vi "S4GUI_003.vi"(7 "Tab ObsEng":enum32{"Obs", "CCD modes", "Guider", "Eng"}(tab)) -> ()   [LabVIEW 2018] (continued)
                n3107 = call-dynamic "Write State Machine.vi"("error in (no error)"=w6764, "State Machine.lvclass"=w6763, "Device in"=w6747) -> ("error out"=w6744:errorcluster, "Device out"=w6746:refnum<class "Channel.lvclass">)  [unwired: 7 in]
              }
            }
            n3108 = case shown="True" w6438 {
              tunnel: w6496 -> [w6710 w6719]
              tunnel: w6495 -> [w6709 w6718]
              tunnel: [w6709 w6717] -> w6494
              tunnel: [w6710 w6716] -> w6493
              frame False {
              }
              frame True {
                n3109 = call-dynamic "Read State Machine.vi"("error in (no error)"=w6718, "Device in"=w6719) -> ("error out"=w6732:errorcluster, "State Machine.lvclass"=w6733:refnum<class "State Machine.lvclass">, "Device out"=w6720:refnum<class "Channel.lvclass">)  [unwired: 7 in]
                n3110 = call-dynamic "Read ref StatesQueue.vi"("error in (no error)"=w6732, "State Machine in"=w6733) -> ("error out"=w6730:errorcluster, "ref StatesQueue"=w6731:refnum<queue>, "State Machine out"=w6727:refnum<class "State Machine.lvclass">)  [unwired: 7 in]
                n3111 = Flush Queue(queue=w6731, error in (no error)=w6730) -> (queue out=w6729:refnum<queue>, error out=w6725:errorcluster)  [unwired: 1 out]
                n3112 = Enqueue Element(queue=w6729, element=u32 300 ("State"), error in (no error)=w6725) -> (queue out=w6714:refnum<queue>, error out=w6712:errorcluster)  [unwired: 1 in, 1 out]
                n3113 = Enqueue Element(queue=w6714, element=u32 305 ("State"), error in (no error)=w6712) -> (queue out=w6713:refnum<queue>, error out=w6711:errorcluster)  [unwired: 1 in, 1 out]
                n3114 = Enqueue Element(queue=w6713, element=u32 60 ("State"), error in (no error)=w6711) -> (queue out=w6728:refnum<queue>, error out=w6726:errorcluster)  [unwired: 1 in, 1 out]
                n3115 = call-dynamic "Write ref StatesQueue.vi"("error in (no error)"=w6726, "ref StatesQueue"=w6728, "State Machine in"=w6727) -> ("error out"=w6723:errorcluster, "State Machine out"=w6724:refnum<class "State Machine.lvclass">)  [unwired: 7 in]
                n3116 = call-dynamic "Write State.vi"("error in (no error)"=w6723, "State"=0, "State Machine in"=w6724) -> ("error out"=w6736:errorcluster, "State Machine out"=w6735:refnum<class "State Machine.lvclass">)  [unwired: 7 in]
                n3117 = call-dynamic "Write State Machine.vi"("error in (no error)"=w6736, "State Machine.lvclass"=w6735, "Device in"=w6720) -> ("error out"=w6717:errorcluster, "Device out"=w6716:refnum<class "Channel.lvclass">)  [unwired: 7 in]
              }
            }
            n3118 = case shown="True" w6439 {
              tunnel: w6446 -> [w6682 w6695]
              tunnel: w6445 -> [w6681 w6694]
              tunnel: [w6681 w6693] -> w6444
              tunnel: [w6682 w6692] -> w6443
              frame False {
              }
              frame True {
                n3119 = call-dynamic "Read State Machine.vi"("error in (no error)"=w6694, "Device in"=w6695) -> ("error out"=w6706:errorcluster, "State Machine.lvclass"=w6691:refnum<class "State Machine.lvclass">, "Device out"=w6696:refnum<class "Channel.lvclass">)  [unwired: 7 in]
                n3120 = call-dynamic "Read ref StatesQueue.vi"("error in (no error)"=w6706, "State Machine in"=w6691) -> ("error out"=w6704:errorcluster, "ref StatesQueue"=w6705:refnum<queue>, "State Machine out"=w6690:refnum<class "State Machine.lvclass">)  [unwired: 7 in]
                n3121 = Flush Queue(queue=w6705, error in (no error)=w6704) -> (queue out=w6703:refnum<queue>, error out=w6700:errorcluster)  [unwired: 1 out]
                n3122 = Enqueue Element(queue=w6703, element=u32 300 ("State"), error in (no error)=w6700) -> (queue out=w6686:refnum<queue>, error out=w6685:errorcluster)  [unwired: 1 in, 1 out]
                n3123 = Enqueue Element(queue=w6686, element=u32 305 ("State"), error in (no error)=w6685) -> (queue out=w6684:refnum<queue>, error out=w6683:errorcluster)  [unwired: 1 in, 1 out]
                n3124 = Enqueue Element(queue=w6684, element=u32 60 ("State"), error in (no error)=w6683) -> (queue out=w6702:refnum<queue>, error out=w6701:errorcluster)  [unwired: 1 in, 1 out]
                n3125 = call-dynamic "Write ref StatesQueue.vi"("error in (no error)"=w6701, "ref StatesQueue"=w6702, "State Machine in"=w6690) -> ("error out"=w6699:errorcluster, "State Machine out"=w6689:refnum<class "State Machine.lvclass">)  [unwired: 7 in]
                n3126 = call-dynamic "Write State.vi"("error in (no error)"=w6699, "State"=0, "State Machine in"=w6689) -> ("error out"=w6708:errorcluster, "State Machine out"=w6688:refnum<class "State Machine.lvclass">)  [unwired: 7 in]
                n3127 = call-dynamic "Write State Machine.vi"("error in (no error)"=w6708, "State Machine.lvclass"=w6688, "Device in"=w6696) -> ("error out"=w6693:errorcluster, "Device out"=w6692:refnum<class "Channel.lvclass">)  [unwired: 7 in]
              }
            }
            n3128 = call-dynamic "Write Channel.vi"("error in (no error)"=w6636, "Channel.lvclass"=w6637, "Acquisition in"=w6651) -> ("error out"=w6679:errorcluster, "Acquisition out"=w6680:refnum<class "Acquisition.lvclass">)  [unwired: 7 in]
            n3129 = call-dynamic "Write Channel.vi"("error in (no error)"=w6546, "Channel.lvclass"=w6548, "Acquisition in"=w6585) -> ("error out"=w6677:errorcluster, "Acquisition out"=w6678:refnum<class "Acquisition.lvclass">)  [unwired: 7 in]
            n3130 = call-dynamic "Write Channel.vi"("error in (no error)"=w6494, "Channel.lvclass"=w6493, "Acquisition in"=w6532) -> ("error out"=w6675:errorcluster, "Acquisition out"=w6676:refnum<class "Acquisition.lvclass">)  [unwired: 7 in]
            n3131 = call-dynamic "Write Channel.vi"("error in (no error)"=w6444, "Channel.lvclass"=w6443, "Acquisition in"=w6492) -> ("error out"=w6673:errorcluster, "Acquisition out"=w6674:refnum<class "Acquisition.lvclass">)  [unwired: 7 in]
          }
        }
        n3132 = call-dynamic "Write AcquisitionA.vi"("error in (no error)"=w5592, "Acquisition.lvclass"=w5593, "S4ACS_GUI in"=w5594) -> ("error out"=w5584:errorcluster, "S4ACS_GUI out"=w5588:refnum<class "S4GUI.lvclass">)  [unwired: 7 in]
        n3133 = call "Write AcquisitionB.vi"("error in (no error)"=w5589, "Acquisition.lvclass"=w5590, "S4ACS_GUI in"=w5588) -> ("error out"=w5583:errorcluster, "S4ACS_GUI out"=w5587:refnum<class "S4GUI.lvclass">)  [unwired: 7 in]
        n3134 = call-dynamic "Write AcquisitionC.vi"("error in (no error)"=w5578, "Acquisition.lvclass"=w5579, "S4ACS_GUI in"=w5587) -> ("error out"=w5582:errorcluster, "S4ACS_GUI out"=w5586:refnum<class "S4GUI.lvclass">)  [unwired: 7 in]
        n3135 = call-dynamic "Write AcquisitionD.vi"("error in (no error)"=w5576, "Acquisition.lvclass"=w5577, "S4ACS_GUI in"=w5586) -> ("error out"=w5581:errorcluster, "S4ACS_GUI out"=w5585:refnum<class "S4GUI.lvclass">)  [unwired: 7 in]
        n3136 = Merge Errors(w5584, w5583, w5582, w5581) -> (w5580:errorcluster)
        n3137 = call "Write cfg file.vi"("error in (no error)"=w5580, "cfg file"="lastsaved.cfg", "S4ACS_GUI in"=w5585) -> ("error out"=w5536:errorcluster, "S4ACS_GUI out"=w5537:refnum<class "S4GUI.lvclass">)  [unwired: 7 in]
        n3138 = disable-structure shown="Enabled" {
          disable-tunnel: w5537 -> [w5598 w5633]
          disable-tunnel: w5536 -> [w5597 w5632]
          disable-tunnel: [w5596 w5633] -> w5535
          disable-tunnel: [w5595 w5632] -> w5534
          frame Disabled {
            # "Este código passou para o evento \"Timeout\" (executa sempre)"
            # "1a vez FOTOM (F)"
            # "1a vez POLAR (F)"
            n3139 = call "Read Instrument.lvclass.vi"("error in (no error)"=w5597, "S4ACS_GUI in"=w5598) -> ("error out"=w5600:errorcluster, "Instrument.lvclass"=w5601:refnum<class "Instrument.lvclass">, "S4ACS_GUI out"=w5596:refnum<class "S4GUI.lvclass">)  [unwired: 7 in]
            n3140 = call-dynamic "Read mode.vi"("error in (no error)"=w5600, "Instrument in"=w5601) -> ("error out"=w5595:errorcluster, "mode"=w5599:bool)  [unwired: 7 in, 1 out]
            n3141 = while {
              tunnel: w5599 -> [w5606]
              shift-right: [w5602] -> _
              shift-left: _ -> [w5605]
              shift-right: [w5603] -> _
              shift-left: _ -> [w5604]
              stop <- TRUE stop-if-true
              # "Valores default para procedimento\nde ajuste de foco do telescópio"
              n3142 = case shown="True" w5606 {
                tunnel: w5605 -> [w5608 w5623]
                tunnel: [w5609 w5622] -> w5602
                tunnel: w5604 -> [w5611 w5621]
                tunnel: [w5610 w5620] -> w5603
                frame True {
                  # "polarimetria"
                  n3143 = case shown="False" w5611 {
                    selector: w5611 -> [w5615 w5619]
                    tunnel: [w5614 w5619] -> w5610
                    tunnel: [FALSE FALSE] -> w5609
                    tunnel: w5608 -> [_ _]
                    frame False {
                      w5612 = 12900
                      n3144 = local write "Start focus"(w5612) -> ()
                      n3145 = local write "Target focus"(w5612) -> ()
                      n3146 = local write "Step focus"(80) -> ()
                      n3147 = local write "#steps"(11) -> ()
                      n3148 = Not(x=w5615) -> (.not. x?=w5614:bool)
                    }
                    frame True {
                    }
                  }
                }
                frame False {
                  # "fotometria"
                  n3149 = case shown="False" w5623 {
                    selector: w5623 -> [w5626 w5631]
                    tunnel: [w5625 w5631] -> w5622
                    tunnel: w5621 -> [_ _]
                    tunnel: [FALSE FALSE] -> w5620
                    frame False {
                      w5624 = 13400
                      n3150 = local write "Start focus"(w5624) -> ()
                      n3151 = local write "Step focus"(100) -> ()
                      n3152 = local write "Target focus"(w5624) -> ()
                      n3153 = local write "#steps"(11) -> ()
                      n3154 = Not(x=w5626) -> (.not. x?=w5625:bool)
                    }
                    frame True {
                    }
                  }
                }
              }
            }
          }
          frame Enabled {
          }
        }
      }
      event "set keywords", "set Observer": Value Change {
        # "SET suffix e publica os outros campos da aba selecionada."
        n3155 = event-data() -> ()  [unwired: 1 in, 1 out]
        n3156 = local read "Tab Acq Type"() -> (w6983:T1)
        n3157 = case shown="\"OBJECT\", Default" w6983 {
          tunnel: ["OBJECT" "FLAT" "FLAT" "DARK" "ZERO" "FOCUS"] -> w6962
          tunnel: [w7064 w7068 w7072 w7076 w7080 w7085] -> w6963
          tunnel: [w7063 w7067 w7071 w7075 w7079 w7084] -> w6957
          tunnel: [w7062 w7066 w7070 w7074 w7078 w7083] -> w6956
          tunnel: [_ _ _ _ _ TRUE] -> _
          frame "OBJECT", Default {
            n3158 = local read "OBJECT Comments"() -> (w7062:string)
            n3159 = local read "Object_obj"() -> (w7064:string)
            n3160 = local read "object suffix"() -> (w7063:string)
          }
          frame "DFLAT" {
            n3161 = local read "DFLAT Comments"() -> (w7066:string)
            n3162 = local read "Object_dflat"() -> (w7068:string)
            n3163 = local read "dflat suffix"() -> (w7067:string)
          }
          frame "SFLAT" {
            n3164 = local read "SFLAT Comments"() -> (w7070:string)
            n3165 = local read "Object_sflat"() -> (w7072:string)
            n3166 = local read "sflat suffix"() -> (w7071:string)
          }
          frame "DARK" {
            n3167 = local read "DARK Comments"() -> (w7074:string)
            n3168 = local read "Object_dark"() -> (w7076:string)
            n3169 = local read "dark suffix"() -> (w7075:string)
          }
          frame "ZERO" {
            n3170 = local read "ZERO Comments"() -> (w7078:string)
            n3171 = local read "Object_zero"() -> (w7080:string)
            n3172 = local read "zero suffix"() -> (w7079:string)
          }
          frame "FOCUS" {
            n3173 = local read "FOCUS Comments"() -> (w7083:string)
            n3174 = local read "Object_focus"() -> (w7085:string)
            n3175 = local read "focus suffix"() -> (w7084:string)
          }
        }
        n3176 = call-dynamic "Write User Event.vi"("error in (no error)"=w6951, "User Event"="SET KEYWORDS CLICKED (Obsever, ProjectID, Object, Comments) ", "S4GUI in"=w6952) -> ("error out"=w6949:errorcluster, "S4GUI out"=w6950:refnum<class "S4GUI.lvclass">)  [unwired: 7 in]
        n3177 = call-dynamic "Read Publisher.lvclass.vi"("error in (no error)"=w6949, "S4GUI in"=w6950) -> ("error out"=w6973:errorcluster, "Publisher.lvclass"=w6969:refnum<class "Publisher.lvclass">, "S4GUI out"=w6974:refnum<class "S4GUI.lvclass">)  [unwired: 7 in]
        n3178 = call-dynamic "Write object.vi"("error in (no error)"=w6973, "object"=w6963, "Publisher in"=w6969) -> ("error out"=w6972:errorcluster, "Publisher out"=w6968:refnum<class "Publisher.lvclass">)  [unwired: 7 in]
        n3179 = call-dynamic "Write obstype.vi"("error in (no error)"=w6972, "obstype"=w6962, "Publisher in"=w6968) -> ("error out"=w6971:errorcluster, "Publisher out"=w6967:refnum<class "Publisher.lvclass">)  [unwired: 7 in]
        n3180 = call-dynamic "Write observer.vi"("error in (no error)"=w6971, "observer"=w6961, "Publisher in"=w6967) -> ("error out"=w6970:errorcluster, "Publisher out"=w6966:refnum<class "Publisher.lvclass">)  [unwired: 7 in]
        n3181 = call-dynamic "Write projid.vi"("error in (no error)"=w6970, "projid"=w6960, "Publisher in"=w6966) -> ("error out"=w6955:errorcluster, "Publisher out"=w6954:refnum<class "Publisher.lvclass">)  [unwired: 7 in]
        n3182 = call-dynamic "Write comments.vi"("error in (no error)"=w6955, "comments"=w6956, "Publisher in"=w6954) -> ("error out"=w6959:errorcluster, "Publisher out"=w6958:refnum<class "Publisher.lvclass">)  [unwired: 7 in]
        n3183 = call-dynamic "Write Publisher.lvclass.vi"("error in (no error)"=w6959, "Publisher.lvclass"=w6958, "S4GUI in"=w6974) -> ("error out"=w6964:errorcluster, "S4GUI out"=w6965:refnum<class "S4GUI.lvclass">)  [unwired: 7 in]
        n3184 = call-dynamic "Read AcquisitionC.vi"("error in (no error)"=w6964, "S4ACS_GUI in"=w6965) -> ("error out"=w6987:errorcluster, "Acquisition.lvclass"=w6988:refnum<class "Acquisition.lvclass">)  [unwired: 7 in, 1 out]
        n3185 = call-dynamic "Read AcquisitionA.vi"("error in (no error)"=w6964, "S4ACS_GUI in"=w6965) -> ("error out"=w6991:errorcluster, "Acquisition.lvclass"=w6992:refnum<class "Acquisition.lvclass">, "S4ACS_GUI out"=w7013:refnum<class "S4GUI.lvclass">)  [unwired: 7 in]
        n3186 = call "Read AcquisitionB.vi"("error in (no error)"=w6964, "S4ACS_GUI in"=w6965) -> ("error out"=w6989:errorcluster, "Acquisition.lvclass"=w6990:refnum<class "Acquisition.lvclass">)  [unwired: 7 in, 1 out]
        n3187 = call-dynamic "Read AcquisitionD.vi"("error in (no error)"=w6964, "S4ACS_GUI in"=w6965) -> ("error out"=w6985:errorcluster, "Acquisition.lvclass"=w6986:refnum<class "Acquisition.lvclass">)  [unwired: 7 in, 1 out]
        n3188 = call-dynamic "Read enabled.vi"("error in (no error)"=w6987, "Server in"=w6988) -> ("error out"=w6977:errorcluster, "enabled"=w6871:bool, "Server out"=w6978:refnum<class "Acquisition.lvclass">)  [unwired: 7 in]
        n3189 = call-dynamic "Read enabled.vi"("error in (no error)"=w6985, "Server in"=w6986) -> ("error out"=w6975:errorcluster, "enabled"=w6845:bool, "Server out"=w6976:refnum<class "Acquisition.lvclass">)  [unwired: 7 in]
        n3190 = call-dynamic "Read enabled.vi"("error in (no error)"=w6989, "Server in"=w6990) -> ("error out"=w6979:errorcluster, "enabled"=w6897:bool, "Server out"=w6980:refnum<class "Acquisition.lvclass">)  [unwired: 7 in]
        n3191 = call-dynamic "Read enabled.vi"("error in (no error)"=w6991, "Server in"=w6992) -> ("error out"=w6981:errorcluster, "enabled"=w6923:bool, "Server out"=w6982:refnum<class "Acquisition.lvclass">)  [unwired: 7 in]
        n3192 = call-dynamic "Read Channel.vi"("error in (no error)"=w6979, "Acquisition in"=w6980) -> ("error out"=w6902:errorcluster, "Channel.lvclass"=w6903:refnum<class "Channel.lvclass">, "Acquisition out"=w6920:refnum<class "Acquisition.lvclass">)  [unwired: 7 in]
        n3193 = call-dynamic "Read Channel.vi"("error in (no error)"=w6975, "Acquisition in"=w6976) -> ("error out"=w6850:errorcluster, "Channel.lvclass"=w6851:refnum<class "Channel.lvclass">, "Acquisition out"=w6870:refnum<class "Acquisition.lvclass">)  [unwired: 7 in]
        n3194 = call-dynamic "Read Channel.vi"("error in (no error)"=w6977, "Acquisition in"=w6978) -> ("error out"=w6876:errorcluster, "Channel.lvclass"=w6877:refnum<class "Channel.lvclass">, "Acquisition out"=w6894:refnum<class "Acquisition.lvclass">)  [unwired: 7 in]
        n3195 = call-dynamic "Read Channel.vi"("error in (no error)"=w6981, "Acquisition in"=w6982) -> ("error out"=w6928:errorcluster, "Channel.lvclass"=w6929:refnum<class "Channel.lvclass">, "Acquisition out"=w6948:refnum<class "Acquisition.lvclass">)  [unwired: 7 in]
        n3196 = To Lower Case(string=w6957) -> (all lower case string=w6984:string)
        n3197 = local read "Filter2"() -> (w6904:u8)
        n3198 = local read "Filter4"() -> (w6852:u8)
        n3199 = local read "Filter3"() -> (w6878:u8)
        n3200 = local read "Filter1"() -> (w6932:u8)
        n3201 = call-dynamic "Write Filter.vi"("error in (no error)"=w6850, "Filter"=w6852, "Channel in"=w6851) -> ("error out"=w6867:errorcluster, "Channel out"=w6856:refnum<class "Channel.lvclass">)  [unwired: 7 in]
        n3202 = call-dynamic "Write Filter.vi"("error in (no error)"=w6902, "Filter"=w6904, "Channel in"=w6903) -> ("error out"=w6919:errorcluster, "Channel out"=w6908:refnum<class "Channel.lvclass">)  [unwired: 7 in]
        n3203 = call-dynamic "Write Filter.vi"("error in (no error)"=w6876, "Filter"=w6878, "Channel in"=w6877) -> ("error out"=w6881:errorcluster, "Channel out"=w6892:refnum<class "Channel.lvclass">)  [unwired: 7 in]
        n3204 = call-dynamic "Write Filter.vi"("error in (no error)"=w6928, "Filter"=w6932, "Channel in"=w6929) -> ("error out"=w6945:errorcluster, "Channel out"=w6944:refnum<class "Channel.lvclass">)  [unwired: 7 in]
        n3205 = call-dynamic "Read Interface.vi"("error in (no error)"=w6867, "Channel in"=w6856) -> ("error out"=w6866:errorcluster, "Interface.lvclass"=w6865:refnum<class "Interface.lvclass">, "Channel out"=w6855:refnum<class "Channel.lvclass">)  [unwired: 7 in]
        n3206 = call-dynamic "Read Interface.vi"("error in (no error)"=w6919, "Channel in"=w6908) -> ("error out"=w6918:errorcluster, "Interface.lvclass"=w6917:refnum<class "Interface.lvclass">, "Channel out"=w6907:refnum<class "Channel.lvclass">)  [unwired: 7 in]
        n3207 = call-dynamic "Read Interface.vi"("error in (no error)"=w6881, "Channel in"=w6892) -> ("error out"=w6882:errorcluster, "Interface.lvclass"=w6883:refnum<class "Interface.lvclass">, "Channel out"=w6893:refnum<class "Channel.lvclass">)  [unwired: 7 in]
        n3208 = call-dynamic "Read Interface.vi"("error in (no error)"=w6945, "Channel in"=w6944) -> ("error out"=w6943:errorcluster, "Interface.lvclass"=w6942:refnum<class "Interface.lvclass">, "Channel out"=w6936:refnum<class "Channel.lvclass">)  [unwired: 7 in]
        n3209 = call-dynamic "Write Suffix.vi"("error in (no error)"=w6943, "Suffix"=w6984, "Interface in"=w6942) -> ("error out"=w6933:errorcluster, "Interface out"=w6937:refnum<class "Interface.lvclass">)  [unwired: 7 in]
        n3210 = call-dynamic "Write Suffix.vi"("error in (no error)"=w6866, "Suffix"=w6984, "Interface in"=w6865) -> ("error out"=w6857:errorcluster, "Interface out"=w6860:refnum<class "Interface.lvclass">)  [unwired: 7 in]
        n3211 = call-dynamic "Write Suffix.vi"("error in (no error)"=w6918, "Suffix"=w6984, "Interface in"=w6917) -> ("error out"=w6909:errorcluster, "Interface out"=w6912:refnum<class "Interface.lvclass">)  [unwired: 7 in]
        n3212 = call-dynamic "Write Suffix.vi"("error in (no error)"=w6882, "Suffix"=w6984, "Interface in"=w6883) -> ("error out"=w6891:errorcluster, "Interface out"=w6888:refnum<class "Interface.lvclass">)  [unwired: 7 in]
        n3213 = call-dynamic "Write ObsType.vi"("error in (no error)"=w6933, "ObsType"=w6962, "Interface in"=w6937) -> ("error out"=w6934:errorcluster, "Interface out"=w6938:refnum<class "Interface.lvclass">)  [unwired: 7 in]
        n3214 = call-dynamic "Write ObsType.vi"("error in (no error)"=w6857, "ObsType"=w6962, "Interface in"=w6860) -> ("error out"=w6858:errorcluster, "Interface out"=w6861:refnum<class "Interface.lvclass">)  [unwired: 7 in]
        n3215 = call-dynamic "Write ObsType.vi"("error in (no error)"=w6909, "ObsType"=w6962, "Interface in"=w6912) -> ("error out"=w6910:errorcluster, "Interface out"=w6913:refnum<class "Interface.lvclass">)  [unwired: 7 in]
        n3216 = call-dynamic "Write ObsType.vi"("error in (no error)"=w6891, "ObsType"=w6962, "Interface in"=w6888) -> ("error out"=w6890:errorcluster, "Interface out"=w6887:refnum<class "Interface.lvclass">)  [unwired: 7 in]
        n3217 = call-dynamic "Write Object.vi"("error in (no error)"=w6934, "Object"=w6963, "Interface in"=w6938) -> ("error out"=w6935:errorcluster, "Interface out"=w6939:refnum<class "Interface.lvclass">)  [unwired: 7 in]
        n3218 = call-dynamic "Write Object.vi"("error in (no error)"=w6910, "Object"=w6963, "Interface in"=w6913) -> ("error out"=w6911:errorcluster, "Interface out"=w6914:refnum<class "Interface.lvclass">)  [unwired: 7 in]
        n3219 = call-dynamic "Write Object.vi"("error in (no error)"=w6858, "Object"=w6963, "Interface in"=w6861) -> ("error out"=w6859:errorcluster, "Interface out"=w6862:refnum<class "Interface.lvclass">)  [unwired: 7 in]
        n3220 = call-dynamic "Write Object.vi"("error in (no error)"=w6890, "Object"=w6963, "Interface in"=w6887) -> ("error out"=w6889:errorcluster, "Interface out"=w6886:refnum<class "Interface.lvclass">)  [unwired: 7 in]
        n3221 = call-dynamic "Write Comments.vi"("error in (no error)"=w6859, "Comments"=w6956, "Interface in"=w6862) -> ("error out"=w6863:errorcluster, "Interface out"=w6864:refnum<class "Interface.lvclass">)  [unwired: 7 in]
        n3222 = call-dynamic "Write Comments.vi"("error in (no error)"=w6911, "Comments"=w6956, "Interface in"=w6914) -> ("error out"=w6915:errorcluster, "Interface out"=w6916:refnum<class "Interface.lvclass">)  [unwired: 7 in]
        n3223 = call-dynamic "Write Comments.vi"("error in (no error)"=w6889, "Comments"=w6956, "Interface in"=w6886) -> ("error out"=w6885:errorcluster, "Interface out"=w6884:refnum<class "Interface.lvclass">)  [unwired: 7 in]
        n3224 = call-dynamic "Write Comments.vi"("error in (no error)"=w6935, "Comments"=w6956, "Interface in"=w6939) -> ("error out"=w6940:errorcluster, "Interface out"=w6941:refnum<class "Interface.lvclass">)  [unwired: 7 in]
        n3225 = call-dynamic "Write Observer.vi"("error in (no error)"=w6863, "Observer"=w6961, "Interface in"=w6864) -> ("error out"=w6849:errorcluster, "Interface out"=w6848:refnum<class "Interface.lvclass">)  [unwired: 7 in]
        n3226 = call-dynamic "Write Observer.vi"("error in (no error)"=w6940, "Observer"=w6961, "Interface in"=w6941) -> ("error out"=w6926:errorcluster, "Interface out"=w6927:refnum<class "Interface.lvclass">)  [unwired: 7 in]
        n3227 = call-dynamic "Write Observer.vi"("error in (no error)"=w6915, "Observer"=w6961, "Interface in"=w6916) -> ("error out"=w6901:errorcluster, "Interface out"=w6900:refnum<class "Interface.lvclass">)  [unwired: 7 in]
        n3228 = call-dynamic "Write Observer.vi"("error in (no error)"=w6885, "Observer"=w6961, "Interface in"=w6884) -> ("error out"=w6875:errorcluster, "Interface out"=w6874:refnum<class "Interface.lvclass">)  [unwired: 7 in]
        n3229 = call-dynamic "Write Project ID.vi"("error in (no error)"=w6875, "Project ID"=w6960, "Interface in"=w6874) -> ("error out"=w6872:errorcluster, "Interface out"=w6873:refnum<class "Interface.lvclass">)  [unwired: 7 in]
        n3230 = call-dynamic "Write Project ID.vi"("error in (no error)"=w6901, "Project ID"=w6960, "Interface in"=w6900) -> ("error out"=w6898:errorcluster, "Interface out"=w6899:refnum<class "Interface.lvclass">)  [unwired: 7 in]
        n3231 = call-dynamic "Write Project ID.vi"("error in (no error)"=w6849, "Project ID"=w6960, "Interface in"=w6848) -> ("error out"=w6846:errorcluster, "Interface out"=w6847:refnum<class "Interface.lvclass">)  [unwired: 7 in]
        n3232 = call-dynamic "Write Project ID.vi"("error in (no error)"=w6926, "Project ID"=w6960, "Interface in"=w6927) -> ("error out"=w6924:errorcluster, "Interface out"=w6925:refnum<class "Interface.lvclass">)  [unwired: 7 in]
        n3233 = call-dynamic "Write Interface.vi"("error in (no error)"=w6898, "Interface.lvclass"=w6899, "Channel in"=w6907) -> ("error out"=w6905:errorcluster, "Channel out"=w6906:refnum<class "Channel.lvclass">)  [unwired: 7 in]
        n3234 = call-dynamic "Write Interface.vi"("error in (no error)"=w6924, "Interface.lvclass"=w6925, "Channel in"=w6936) -> ("error out"=w6930:errorcluster, "Channel out"=w6931:refnum<class "Channel.lvclass">)  [unwired: 7 in]
        n3235 = call-dynamic "Write Interface.vi"("error in (no error)"=w6872, "Interface.lvclass"=w6873, "Channel in"=w6893) -> ("error out"=w6879:errorcluster, "Channel out"=w6880:refnum<class "Channel.lvclass">)  [unwired: 7 in]
        n3236 = call-dynamic "Write Interface.vi"("error in (no error)"=w6846, "Interface.lvclass"=w6847, "Channel in"=w6855) -> ("error out"=w6853:errorcluster, "Channel out"=w6854:refnum<class "Channel.lvclass">)  [unwired: 7 in]
        n3237 = case shown="True" w6897 {
          tunnel: [w7038 w7049] -> w6922
          tunnel: [w7039 w7048] -> w6921
          tunnel: w6906 -> [w7039 w7041]
          tunnel: w6905 -> [w7038 w7040]
          frame False {
          }
          frame True {
            # "command SET SUFFIX"
            n3238 = call-dynamic "Read State Machine.vi"("error in (no error)"=w7040, "Device in"=w7041) -> ("error out"=w7042:errorcluster, "State Machine.lvclass"=w7046:refnum<class "State Machine.lvclass">, "Device out"=w7045:refnum<class "Channel.lvclass">)  [unwired: 7 in]
            n3239 = call-dynamic "Write State.vi"("error in (no error)"=w7042, "State"=300, "State Machine in"=w7046) -> ("error out"=w7043:errorcluster, "State Machine out"=w7047:refnum<class "State Machine.lvclass">)  [unwired: 7 in]
            n3240 = call-dynamic "Write State Machine.vi"("error in (no error)"=w7043, "State Machine.lvclass"=w7047, "Device in"=w7045) -> ("error out"=w7049:errorcluster, "Device out"=w7048:refnum<class "Channel.lvclass">)  [unwired: 7 in]
          }
        }
        n3241 = case shown="True" w6923 {
          tunnel: [w7051 w7055] -> w6947
          tunnel: [w7050 w7054] -> w6946
          tunnel: w6931 -> [w7051 w7053]
          tunnel: w6930 -> [w7050 w7052]
          frame False {
          }
          frame True {
            # "command SET SUFFIX"
            n3242 = call-dynamic "Read State Machine.vi"("error in (no error)"=w7052, "Device in"=w7053) -> ("error out"=w7061:errorcluster, "State Machine.lvclass"=w7057:refnum<class "State Machine.lvclass">, "Device out"=w7058:refnum<class "Channel.lvclass">)  [unwired: 7 in]
            n3243 = call-dynamic "Write State.vi"("error in (no error)"=w7061, "State"=300, "State Machine in"=w7057) -> ("error out"=w7060:errorcluster, "State Machine out"=w7056:refnum<class "State Machine.lvclass">)  [unwired: 7 in]
            n3244 = call-dynamic "Write State Machine.vi"("error in (no error)"=w7060, "State Machine.lvclass"=w7056, "Device in"=w7058) -> ("error out"=w7054:errorcluster, "Device out"=w7055:refnum<class "Channel.lvclass">)  [unwired: 7 in]
          }
        }
        n3245 = case shown="True" w6871 {
          tunnel: [w7026 w7037] -> w6896
          tunnel: [w7027 w7036] -> w6895
          tunnel: w6880 -> [w7027 w7029]
          tunnel: w6879 -> [w7026 w7028]
          frame False {
          }
          frame True {
            # "command SET SUFFIX"
            n3246 = call-dynamic "Read State Machine.vi"("error in (no error)"=w7028, "Device in"=w7029) -> ("error out"=w7030:errorcluster, "State Machine.lvclass"=w7034:refnum<class "State Machine.lvclass">, "Device out"=w7033:refnum<class "Channel.lvclass">)  [unwired: 7 in]
            n3247 = call-dynamic "Write State.vi"("error in (no error)"=w7030, "State"=300, "State Machine in"=w7034) -> ("error out"=w7031:errorcluster, "State Machine out"=w7035:refnum<class "State Machine.lvclass">)  [unwired: 7 in]
            n3248 = call-dynamic "Write State Machine.vi"("error in (no error)"=w7031, "State Machine.lvclass"=w7035, "Device in"=w7033) -> ("error out"=w7037:errorcluster, "Device out"=w7036:refnum<class "Channel.lvclass">)  [unwired: 7 in]
          }
        }
        n3249 = case shown="True" w6845 {
          tunnel: [w7015 w7019] -> w6869
          tunnel: [w7014 w7018] -> w6868
          tunnel: w6854 -> [w7015 w7017]
          tunnel: w6853 -> [w7014 w7016]
          frame False {
          }
          frame True {
            # "command SET SUFFIX"
            n3250 = call-dynamic "Read State Machine.vi"("error in (no error)"=w7016, "Device in"=w7017) -> ("error out"=w7025:errorcluster, "State Machine.lvclass"=w7021:refnum<class "State Machine.lvclass">, "Device out"=w7022:refnum<class "Channel.lvclass">)  [unwired: 7 in]
            n3251 = call-dynamic "Write State.vi"("error in (no error)"=w7025, "State"=300, "State Machine in"=w7021) -> ("error out"=w7024:errorcluster, "State Machine out"=w7020:refnum<class "State Machine.lvclass">)  [unwired: 7 in]
            n3252 = call-dynamic "Write State Machine.vi"("error in (no error)"=w7024, "State Machine.lvclass"=w7020, "Device in"=w7022) -> ("error out"=w7018:errorcluster, "Device out"=w7019:refnum<class "Channel.lvclass">)  [unwired: 7 in]
          }
        }
        n3253 = call-dynamic "Write Channel.vi"("error in (no error)"=w6946, "Channel.lvclass"=w6947, "Acquisition in"=w6948) -> ("error out"=w7011:errorcluster, "Acquisition out"=w7012:refnum<class "Acquisition.lvclass">)  [unwired: 7 in]
        n3254 = call-dynamic "Write Channel.vi"("error in (no error)"=w6922, "Channel.lvclass"=w6921, "Acquisition in"=w6920) -> ("error out"=w7006:errorcluster, "Acquisition out"=w7007:refnum<class "Acquisition.lvclass">)  [unwired: 7 in]
        n3255 = call-dynamic "Write Channel.vi"("error in (no error)"=w6896, "Channel.lvclass"=w6895, "Acquisition in"=w6894) -> ("error out"=w6995:errorcluster, "Acquisition out"=w6996:refnum<class "Acquisition.lvclass">)  [unwired: 7 in]
        n3256 = call-dynamic "Write Channel.vi"("error in (no error)"=w6868, "Channel.lvclass"=w6869, "Acquisition in"=w6870) -> ("error out"=w6993:errorcluster, "Acquisition out"=w6994:refnum<class "Acquisition.lvclass">)  [unwired: 7 in]
        n3257 = call-dynamic "Write AcquisitionA.vi"("error in (no error)"=w7011, "Acquisition.lvclass"=w7012, "S4ACS_GUI in"=w7013) -> ("error out"=w7001:errorcluster, "S4ACS_GUI out"=w7005:refnum<class "S4GUI.lvclass">)  [unwired: 7 in]
        n3258 = call "Write AcquisitionB.vi"("error in (no error)"=w7006, "Acquisition.lvclass"=w7007, "S4ACS_GUI in"=w7005) -> ("error out"=w7000:errorcluster, "S4ACS_GUI out"=w7004:refnum<class "S4GUI.lvclass">)  [unwired: 7 in]
        n3259 = call-dynamic "Write AcquisitionC.vi"("error in (no error)"=w6995, "Acquisition.lvclass"=w6996, "S4ACS_GUI in"=w7004) -> ("error out"=w6999:errorcluster, "S4ACS_GUI out"=w7003:refnum<class "S4GUI.lvclass">)  [unwired: 7 in]
        n3260 = call-dynamic "Write AcquisitionD.vi"("error in (no error)"=w6993, "Acquisition.lvclass"=w6994, "S4ACS_GUI in"=w7003) -> ("error out"=w6998:errorcluster, "S4ACS_GUI out"=w7002:refnum<class "S4GUI.lvclass">)  [unwired: 7 in]
        n3261 = Merge Errors(w7001, w7000, w6999, w6998) -> (w6997:errorcluster)
        n3262 = call "Write cfg file.vi"("error in (no error)"=w6997, "cfg file"="lastsaved.cfg", "S4ACS_GUI in"=w7002) -> ("error out"=w7009:errorcluster, "S4ACS_GUI out"=w7008:refnum<class "S4GUI.lvclass">)  [unwired: 7 in]
      }
      event "Object_sflat", "Object_dark", "Object_zero", "Object_dflat", "Object_focus", "Object_obj": Value Change {
        n3263 = event-data() -> ("NewVal"=w7087:string)  [unwired: 1 in, 5 out]
        n3264 = stacked-sequence {
          seq-local: [w7117 _ _ _] -> [_ w7181 _ _]
          seq-local: [w7116 _ _ _] -> [_ w7180 _ _]
          seq-local: [_ w7179 _ _] -> [_ _ w7230 _]
          seq-local: [_ w7178 _ _] -> [_ _ w7229 _]
          seq-local: [_ _ w7228 _] -> [_ _ _ w7279]
          seq-local: [_ _ w7227 _] -> [_ _ _ w7278]
          tunnel: w7094 -> [w7129 _ _ _]
          tunnel: w7095 -> [w7128 _ _ _]
          tunnel: [_ _ _ w7277] -> w7089
          tunnel: [_ _ _ w7276] -> w7088
          tunnel: w7093 -> [w7115 w7177 w7226 w7275]
          tunnel: w7092 -> [w7114 w7176 w7212 w7261]
          tunnel: w7090 -> [w7113 w7162 w7211 w7260]
          tunnel: w7087 -> [w7112 w7161 w7210 w7259]
          tunnel: w7091 -> [w7111 w7160 w7209 w7258]
          frame #0 {
            # "observer"
            # "comment"
            # "object"
            # "suffix"
            # "obsType"
            n3265 = call-dynamic "Read AcquisitionA.vi"("error in (no error)"=w7129, "S4ACS_GUI in"=w7128) -> ("error out"=w7127:errorcluster, "Acquisition.lvclass"=w7126:refnum<class "Acquisition.lvclass">, "S4ACS_GUI out"=w7121:refnum<class "S4GUI.lvclass">)  [unwired: 7 in]
            n3266 = call-dynamic "Read Channel.vi"("error in (no error)"=w7127, "Acquisition in"=w7126) -> ("error out"=w7097:errorcluster, "Channel.lvclass"=w7100:refnum<class "Channel.lvclass">, "Acquisition out"=w7120:refnum<class "Acquisition.lvclass">)  [unwired: 7 in]
            n3267 = local read "Filter1"() -> (w7098:u8)
            n3268 = call-dynamic "Write Filter.vi"("error in (no error)"=w7097, "Filter"=w7098, "Channel in"=w7100) -> ("error out"=w7096:errorcluster, "Channel out"=w7099:refnum<class "Channel.lvclass">)  [unwired: 7 in]
            n3269 = call-dynamic "Read Interface.vi"("error in (no error)"=w7096, "Channel in"=w7099) -> ("error out"=w7107:errorcluster, "Interface.lvclass"=w7108:refnum<class "Interface.lvclass">, "Channel out"=w7125:refnum<class "Channel.lvclass">)  [unwired: 7 in]
            n3270 = call-dynamic "Write Suffix.vi"("error in (no error)"=w7107, "Suffix"=w7115, "Interface in"=w7108) -> ("error out"=w7132:errorcluster, "Interface out"=w7124:refnum<class "Interface.lvclass">)  [unwired: 7 in]
            n3271 = call-dynamic "Write ObsType.vi"("error in (no error)"=w7132, "ObsType"=w7113, "Interface in"=w7124) -> ("error out"=w7131:errorcluster, "Interface out"=w7123:refnum<class "Interface.lvclass">)  [unwired: 7 in]
            n3272 = call-dynamic "Write Object.vi"("error in (no error)"=w7131, "Object"=w7112, "Interface in"=w7123) -> ("error out"=w7130:errorcluster, "Interface out"=w7122:refnum<class "Interface.lvclass">)  [unwired: 7 in]
            n3273 = call-dynamic "Write Comments.vi"("error in (no error)"=w7130, "Comments"=w7114, "Interface in"=w7122) -> ("error out"=w7110:errorcluster, "Interface out"=w7109:refnum<class "Interface.lvclass">)  [unwired: 7 in]
            n3274 = call-dynamic "Write Observer.vi"("error in (no error)"=w7110, "Observer"=w7111, "Interface in"=w7109) -> ("error out"=w7105:errorcluster, "Interface out"=w7106:refnum<class "Interface.lvclass">)  [unwired: 7 in]
            n3275 = call-dynamic "Write Interface.vi"("error in (no error)"=w7105, "Interface.lvclass"=w7106, "Channel in"=w7125) -> ("error out"=w7102:errorcluster, "Channel out"=w7104:refnum<class "Channel.lvclass">)  [unwired: 7 in]
            n3276 = disable-structure shown="Enabled" {
              disable-tunnel: w7104 -> [w7142 w7144]
              disable-tunnel: [w7140 w7144] -> w7103
              disable-tunnel: w7102 -> [w7139 w7143]
              disable-tunnel: [w7134 w7143] -> w7101
              frame Disabled {
                n3277 = call-dynamic "Read State Machine.vi"("error in (no error)"=w7139, "Device in"=w7142) -> ("error out"=w7138:errorcluster, "State Machine.lvclass"=w7136:refnum<class "State Machine.lvclass">, "Device out"=w7141:refnum<class "Channel.lvclass">)  [unwired: 7 in]
                n3278 = call "Next State.vi"("error in (no error)"=w7138, "New_State"=12, "State Machine in"=w7136) -> ("error out"=w7137:errorcluster, "State Machine out"=w7135:refnum<class "State Machine.lvclass">)  [unwired: 7 in]
                n3279 = call-dynamic "Write State Machine.vi"("error in (no error)"=w7137, "State Machine.lvclass"=w7135, "Device in"=w7141) -> ("error out"=w7134:errorcluster, "Device out"=w7140:refnum<class "Channel.lvclass">)  [unwired: 7 in]
              }
              frame Enabled {
              }
            }
            n3280 = call-dynamic "Write Channel.vi"("error in (no error)"=w7101, "Channel.lvclass"=w7103, "Acquisition in"=w7120) -> ("error out"=w7118:errorcluster, "Acquisition out"=w7119:refnum<class "Acquisition.lvclass">)  [unwired: 7 in]
            n3281 = call-dynamic "Write AcquisitionA.vi"("error in (no error)"=w7118, "Acquisition.lvclass"=w7119, "S4ACS_GUI in"=w7121) -> ("error out"=w7116:errorcluster, "S4ACS_GUI out"=w7117:refnum<class "S4GUI.lvclass">)  [unwired: 7 in]
          }
          frame #1 {
            # "object"
            # "suffix"
            # "obsType"
            n3282 = call "Read AcquisitionB.vi"("error in (no error)"=w7180, "S4ACS_GUI in"=w7181) -> ("error out"=w7166:errorcluster, "Acquisition.lvclass"=w7167:refnum<class "Acquisition.lvclass">, "S4ACS_GUI out"=w7172:refnum<class "S4GUI.lvclass">)  [unwired: 7 in]
            n3283 = call-dynamic "Read Channel.vi"("error in (no error)"=w7166, "Acquisition in"=w7167) -> ("error out"=w7146:errorcluster, "Channel.lvclass"=w7148:refnum<class "Channel.lvclass">, "Acquisition out"=w7173:refnum<class "Acquisition.lvclass">)  [unwired: 7 in]
            n3284 = local read "Filter2"() -> (w7149:u8)
            n3285 = call-dynamic "Write Filter.vi"("error in (no error)"=w7146, "Filter"=w7149, "Channel in"=w7148) -> ("error out"=w7145:errorcluster, "Channel out"=w7147:refnum<class "Channel.lvclass">)  [unwired: 7 in]
            n3286 = call-dynamic "Read Interface.vi"("error in (no error)"=w7145, "Channel in"=w7147) -> ("error out"=w7154:errorcluster, "Interface.lvclass"=w7155:refnum<class "Interface.lvclass">, "Channel out"=w7168:refnum<class "Channel.lvclass">)  [unwired: 7 in]
            n3287 = call-dynamic "Write Suffix.vi"("error in (no error)"=w7154, "Suffix"=w7177, "Interface in"=w7155) -> ("error out"=w7163:errorcluster, "Interface out"=w7169:refnum<class "Interface.lvclass">)  [unwired: 7 in]
            n3288 = call-dynamic "Write ObsType.vi"("error in (no error)"=w7163, "ObsType"=w7162, "Interface in"=w7169) -> ("error out"=w7164:errorcluster, "Interface out"=w7170:refnum<class "Interface.lvclass">)  [unwired: 7 in]
            n3289 = call-dynamic "Write Object.vi"("error in (no error)"=w7164, "Object"=w7161, "Interface in"=w7170) -> ("error out"=w7165:errorcluster, "Interface out"=w7171:refnum<class "Interface.lvclass">)  [unwired: 7 in]
            n3290 = call-dynamic "Write Comments.vi"("error in (no error)"=w7165, "Comments"=w7176, "Interface in"=w7171) -> ("error out"=w7157:errorcluster, "Interface out"=w7156:refnum<class "Interface.lvclass">)  [unwired: 7 in]
            n3291 = call-dynamic "Write Observer.vi"("error in (no error)"=w7157, "Observer"=w7160, "Interface in"=w7156) -> ("error out"=w7158:errorcluster, "Interface out"=w7159:refnum<class "Interface.lvclass">)  [unwired: 7 in]
            n3292 = call-dynamic "Write Interface.vi"("error in (no error)"=w7158, "Interface.lvclass"=w7159, "Channel in"=w7168) -> ("error out"=w7152:errorcluster, "Channel out"=w7153:refnum<class "Channel.lvclass">)  [unwired: 7 in]
            n3293 = disable-structure shown="Enabled" {
              disable-tunnel: w7153 -> [w7186 w7193]
              disable-tunnel: w7152 -> [w7185 w7192]
              disable-tunnel: [w7183 w7193] -> w7151
              disable-tunnel: [w7182 w7192] -> w7150
              frame Disabled {
                n3294 = call-dynamic "Read State Machine.vi"("error in (no error)"=w7185, "Device in"=w7186) -> ("error out"=w7191:errorcluster, "State Machine.lvclass"=w7189:refnum<class "State Machine.lvclass">, "Device out"=w7184:refnum<class "Channel.lvclass">)  [unwired: 7 in]
                n3295 = call "Next State.vi"("error in (no error)"=w7191, "New_State"=12, "State Machine in"=w7189) -> ("error out"=w7190:errorcluster, "State Machine out"=w7188:refnum<class "State Machine.lvclass">)  [unwired: 7 in]
                n3296 = call-dynamic "Write State Machine.vi"("error in (no error)"=w7190, "State Machine.lvclass"=w7188, "Device in"=w7184) -> ("error out"=w7182:errorcluster, "Device out"=w7183:refnum<class "Channel.lvclass">)  [unwired: 7 in]
              }
              frame Enabled {
              }
            }
            n3297 = call-dynamic "Write Channel.vi"("error in (no error)"=w7150, "Channel.lvclass"=w7151, "Acquisition in"=w7173) -> ("error out"=w7175:errorcluster, "Acquisition out"=w7174:refnum<class "Acquisition.lvclass">)  [unwired: 7 in]
            n3298 = call "Write AcquisitionB.vi"("error in (no error)"=w7175, "Acquisition.lvclass"=w7174, "S4ACS_GUI in"=w7172) -> ("error out"=w7178:errorcluster, "S4ACS_GUI out"=w7179:refnum<class "S4GUI.lvclass">)  [unwired: 7 in]
          }
          frame #2 {
            # "object"
            # "suffix"
            # "obsType"
            n3299 = call-dynamic "Read AcquisitionC.vi"("error in (no error)"=w7229, "S4ACS_GUI in"=w7230) -> ("error out"=w7222:errorcluster, "Acquisition.lvclass"=w7221:refnum<class "Acquisition.lvclass">, "S4ACS_GUI out"=w7216:refnum<class "S4GUI.lvclass">)  [unwired: 7 in]
            n3300 = call-dynamic "Read Channel.vi"("error in (no error)"=w7222, "Acquisition in"=w7221) -> ("error out"=w7195:errorcluster, "Channel.lvclass"=w7197:refnum<class "Channel.lvclass">, "Acquisition out"=w7215:refnum<class "Acquisition.lvclass">)  [unwired: 7 in]
            n3301 = local read "Filter3"() -> (w7198:u8)
            n3302 = call-dynamic "Write Filter.vi"("error in (no error)"=w7195, "Filter"=w7198, "Channel in"=w7197) -> ("error out"=w7194:errorcluster, "Channel out"=w7196:refnum<class "Channel.lvclass">)  [unwired: 7 in]
            n3303 = call-dynamic "Read Interface.vi"("error in (no error)"=w7194, "Channel in"=w7196) -> ("error out"=w7207:errorcluster, "Interface.lvclass"=w7208:refnum<class "Interface.lvclass">, "Channel out"=w7220:refnum<class "Channel.lvclass">)  [unwired: 7 in]
            n3304 = call-dynamic "Write Suffix.vi"("error in (no error)"=w7207, "Suffix"=w7226, "Interface in"=w7208) -> ("error out"=w7225:errorcluster, "Interface out"=w7219:refnum<class "Interface.lvclass">)  [unwired: 7 in]
            n3305 = call-dynamic "Write ObsType.vi"("error in (no error)"=w7225, "ObsType"=w7211, "Interface in"=w7219) -> ("error out"=w7224:errorcluster, "Interface out"=w7218:refnum<class "Interface.lvclass">)  [unwired: 7 in]
            n3306 = call-dynamic "Write Object.vi"("error in (no error)"=w7224, "Object"=w7210, "Interface in"=w7218) -> ("error out"=w7223:errorcluster, "Interface out"=w7217:refnum<class "Interface.lvclass">)  [unwired: 7 in]
            n3307 = call-dynamic "Write Comments.vi"("error in (no error)"=w7223, "Comments"=w7212, "Interface in"=w7217) -> ("error out"=w7204:errorcluster, "Interface out"=w7203:refnum<class "Interface.lvclass">)  [unwired: 7 in]
            n3308 = call-dynamic "Write Observer.vi"("error in (no error)"=w7204, "Observer"=w7209, "Interface in"=w7203) -> ("error out"=w7205:errorcluster, "Interface out"=w7206:refnum<class "Interface.lvclass">)  [unwired: 7 in]
            n3309 = call-dynamic "Write Interface.vi"("error in (no error)"=w7205, "Interface.lvclass"=w7206, "Channel in"=w7220) -> ("error out"=w7201:errorcluster, "Channel out"=w7202:refnum<class "Channel.lvclass">)  [unwired: 7 in]
            n3310 = disable-structure shown="Enabled" {
              disable-tunnel: w7202 -> [w7237 w7242]
              disable-tunnel: w7201 -> [w7236 w7241]
              disable-tunnel: [w7234 w7242] -> w7200
              disable-tunnel: [w7231 w7241] -> w7199
              frame Disabled {
                n3311 = call-dynamic "Read State Machine.vi"("error in (no error)"=w7236, "Device in"=w7237) -> ("error out"=w7240:errorcluster, "State Machine.lvclass"=w7233:refnum<class "State Machine.lvclass">, "Device out"=w7235:refnum<class "Channel.lvclass">)  [unwired: 7 in]
                n3312 = call "Next State.vi"("error in (no error)"=w7240, "New_State"=12, "State Machine in"=w7233) -> ("error out"=w7239:errorcluster, "State Machine out"=w7232:refnum<class "State Machine.lvclass">)  [unwired: 7 in]
                n3313 = call-dynamic "Write State Machine.vi"("error in (no error)"=w7239, "State Machine.lvclass"=w7232, "Device in"=w7235) -> ("error out"=w7231:errorcluster, "Device out"=w7234:refnum<class "Channel.lvclass">)  [unwired: 7 in]
              }
              frame Enabled {
              }
            }
            n3314 = call-dynamic "Write Channel.vi"("error in (no error)"=w7199, "Channel.lvclass"=w7200, "Acquisition in"=w7215) -> ("error out"=w7213:errorcluster, "Acquisition out"=w7214:refnum<class "Acquisition.lvclass">)  [unwired: 7 in]
            n3315 = call-dynamic "Write AcquisitionC.vi"("error in (no error)"=w7213, "Acquisition.lvclass"=w7214, "S4ACS_GUI in"=w7216) -> ("error out"=w7227:errorcluster, "S4ACS_GUI out"=w7228:refnum<class "S4GUI.lvclass">)  [unwired: 7 in]
          }
          frame #3 {
            # "object"
            # "suffix"
            # "obsType"
            n3316 = call-dynamic "Read AcquisitionD.vi"("error in (no error)"=w7278, "S4ACS_GUI in"=w7279) -> ("error out"=w7271:errorcluster, "Acquisition.lvclass"=w7270:refnum<class "Acquisition.lvclass">, "S4ACS_GUI out"=w7265:refnum<class "S4GUI.lvclass">)  [unwired: 7 in]
            n3317 = call-dynamic "Read Channel.vi"("error in (no error)"=w7271, "Acquisition in"=w7270) -> ("error out"=w7244:errorcluster, "Channel.lvclass"=w7246:refnum<class "Channel.lvclass">, "Acquisition out"=w7264:refnum<class "Acquisition.lvclass">)  [unwired: 7 in]
            n3318 = local read "Filter4"() -> (w7247:u8)
            n3319 = call-dynamic "Write Filter.vi"("error in (no error)"=w7244, "Filter"=w7247, "Channel in"=w7246) -> ("error out"=w7243:errorcluster, "Channel out"=w7245:refnum<class "Channel.lvclass">)  [unwired: 7 in]
            n3320 = call-dynamic "Read Interface.vi"("error in (no error)"=w7243, "Channel in"=w7245) -> ("error out"=w7256:errorcluster, "Interface.lvclass"=w7257:refnum<class "Interface.lvclass">, "Channel out"=w7269:refnum<class "Channel.lvclass">)  [unwired: 7 in]
            n3321 = call-dynamic "Write Suffix.vi"("error in (no error)"=w7256, "Suffix"=w7275, "Interface in"=w7257) -> ("error out"=w7274:errorcluster, "Interface out"=w7268:refnum<class "Interface.lvclass">)  [unwired: 7 in]
            n3322 = call-dynamic "Write ObsType.vi"("error in (no error)"=w7274, "ObsType"=w7260, "Interface in"=w7268) -> ("error out"=w7273:errorcluster, "Interface out"=w7267:refnum<class "Interface.lvclass">)  [unwired: 7 in]
            n3323 = call-dynamic "Write Object.vi"("error in (no error)"=w7273, "Object"=w7259, "Interface in"=w7267) -> ("error out"=w7272:errorcluster, "Interface out"=w7266:refnum<class "Interface.lvclass">)  [unwired: 7 in]
            n3324 = call-dynamic "Write Comments.vi"("error in (no error)"=w7272, "Comments"=w7261, "Interface in"=w7266) -> ("error out"=w7255:errorcluster, "Interface out"=w7254:refnum<class "Interface.lvclass">)  [unwired: 7 in]
            n3325 = call-dynamic "Write Observer.vi"("error in (no error)"=w7255, "Observer"=w7258, "Interface in"=w7254) -> ("error out"=w7253:errorcluster, "Interface out"=w7252:refnum<class "Interface.lvclass">)  [unwired: 7 in]
            n3326 = call-dynamic "Write Interface.vi"("error in (no error)"=w7253, "Interface.lvclass"=w7252, "Channel in"=w7269) -> ("error out"=w7249:errorcluster, "Channel out"=w7251:refnum<class "Channel.lvclass">)  [unwired: 7 in]
            n3327 = disable-structure shown="Enabled" {
              disable-tunnel: w7251 -> [w7286 w7291]
              disable-tunnel: [w7284 w7291] -> w7250
              disable-tunnel: w7249 -> [w7283 w7290]
              disable-tunnel: [w7282 w7290] -> w7248
              frame Disabled {
                n3328 = call-dynamic "Read State Machine.vi"("error in (no error)"=w7283, "Device in"=w7286) -> ("error out"=w7289:errorcluster, "State Machine.lvclass"=w7281:refnum<class "State Machine.lvclass">, "Device out"=w7285:refnum<class "Channel.lvclass">)  [unwired: 7 in]
                n3329 = call "Next State.vi"("error in (no error)"=w7289, "New_State"=12, "State Machine in"=w7281) -> ("error out"=w7288:errorcluster, "State Machine out"=w7280:refnum<class "State Machine.lvclass">)  [unwired: 7 in]
                n3330 = call-dynamic "Write State Machine.vi"("error in (no error)"=w7288, "State Machine.lvclass"=w7280, "Device in"=w7285) -> ("error out"=w7282:errorcluster, "Device out"=w7284:refnum<class "Channel.lvclass">)  [unwired: 7 in]
              }
              frame Enabled {
              }
            }
            n3331 = call-dynamic "Write Channel.vi"("error in (no error)"=w7248, "Channel.lvclass"=w7250, "Acquisition in"=w7264) -> ("error out"=w7262:errorcluster, "Acquisition out"=w7263:refnum<class "Acquisition.lvclass">)  [unwired: 7 in]
            n3332 = call-dynamic "Write AcquisitionD.vi"("error in (no error)"=w7262, "Acquisition.lvclass"=w7263, "S4ACS_GUI in"=w7265) -> ("error out"=w7276:errorcluster, "S4ACS_GUI out"=w7277:refnum<class "S4GUI.lvclass">)  [unwired: 7 in]
          }
        }
      }
      event "DFLAT Comments", "SFLAT Comments", "DARK Comments", "ZERO Comments", "FOCUS Comments", "OBJECT Comments": Value Change {
        n3333 = event-data() -> ("NewVal"=w7292:string)  [unwired: 1 in, 5 out]
        n3334 = disable-structure shown="Enabled" {
          disable-tunnel: w7300 -> [w7309 w7483]
          disable-tunnel: w7299 -> [w7308 w7482]
          disable-tunnel: w7298 -> [w7307 _]
          disable-tunnel: w7297 -> [w7306 _]
          disable-tunnel: w7296 -> [w7305 _]
          disable-tunnel: w7295 -> [w7304 _]
          disable-tunnel: [w7303 w7483] -> w7294
          disable-tunnel: [w7302 w7482] -> w7293
          disable-tunnel: w7292 -> [w7301 _]
          frame Disabled {
            n3335 = stacked-sequence {
              seq-local: [w7337 _ _ _] -> [_ w7395 _ _]
              seq-local: [w7336 _ _ _] -> [_ w7394 _ _]
              seq-local: [_ w7393 _ _] -> [_ _ w7438 _]
              seq-local: [_ w7392 _ _] -> [_ _ w7437 _]
              seq-local: [_ _ w7436 _] -> [_ _ _ w7481]
              seq-local: [_ _ w7435 _] -> [_ _ _ w7480]
              tunnel: w7308 -> [w7349 _ _ _]
              tunnel: w7309 -> [w7348 _ _ _]
              tunnel: [_ _ _ w7479] -> w7303
              tunnel: [_ _ _ w7478] -> w7302
              tunnel: w7306 -> [w7335 w7391 w7434 w7477]
              tunnel: w7301 -> [w7334 w7390 w7420 w7463]
              tunnel: w7304 -> [w7333 w7376 w7419 w7462]
              tunnel: w7307 -> [w7332 w7375 w7418 w7461]
              tunnel: w7305 -> [w7331 w7374 w7417 w7460]
              frame #0 {
                # "observer"
                # "comment"
                # "object"
                # "suffix"
                # "obsType"
                n3336 = call-dynamic "Read AcquisitionA.vi"("error in (no error)"=w7349, "S4ACS_GUI in"=w7348) -> ("error out"=w7347:errorcluster, "Acquisition.lvclass"=w7346:refnum<class "Acquisition.lvclass">, "S4ACS_GUI out"=w7341:refnum<class "S4GUI.lvclass">)  [unwired: 7 in]
                n3337 = call-dynamic "Read Channel.vi"("error in (no error)"=w7347, "Acquisition in"=w7346) -> ("error out"=w7311:errorcluster, "Channel.lvclass"=w7314:refnum<class "Channel.lvclass">, "Acquisition out"=w7340:refnum<class "Acquisition.lvclass">)  [unwired: 7 in]
                n3338 = local read "Filter1"() -> (w7312:u8)
                n3339 = call-dynamic "Write Filter.vi"("error in (no error)"=w7311, "Filter"=w7312, "Channel in"=w7314) -> ("error out"=w7310:errorcluster, "Channel out"=w7313:refnum<class "Channel.lvclass">)  [unwired: 7 in]
